vi "Initialize.vi"(7 "Serial Configuration":T1={"Baud Rate"=9600, "Flow Control"=0, "Parity"=0, "Stop Bits"=10, "Data Bits"=8} {"Stop Bits" items=["1.0"=10, "1.5"=15, "2.0"=20]; "Parity" items=["None", "Odd", "Even", "Mark", "Space"]; "Flow Control" items=["None", "XON/XOFF", "RTS/CTS"]}, 8 "error in (no error)":errorcluster, 9 "Reset (True)":bool=TRUE, 10 "ID Query (True)":bool=TRUE, 11 "VISA resource name":refnum<visa-resource-name>) -> (0 "error out":errorcluster, 3 "VISA resource name out":refnum<visa-resource-name>)   [LabVIEW 2020, in "Keithley DMM6500 DAQ6500 Series.lvlib"]
doc: "Establishes communication with the instrument and optionally performs an instrument identification query and/or an instrument reset. It also places the instrument in a default state needed for other instrument driver operations. Therefore, call this VI before calling other instrument driver VIs for this instrument. Generally, you need to call the <b>Initialize</b> VI only once at the beginning of an application."
uses:
  <instrlib>/Keithley DMM6500 DAQ6500 Series/Keithley DMM6500 DAQ6500 Series.lvlib
panel:
  # "(c) 2018-2022 National Instruments.  ALL RIGHTS RESERVED."
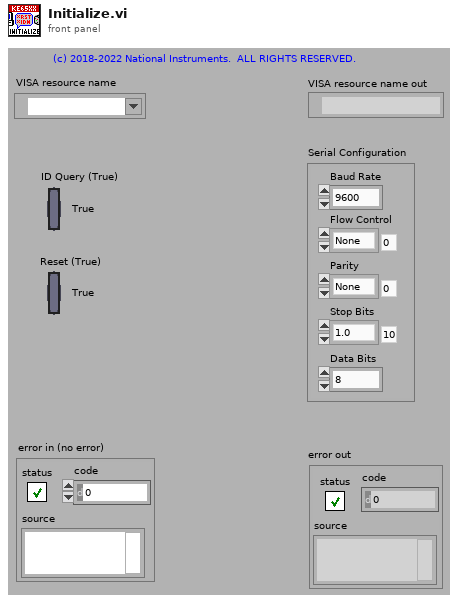
[diagram p1: front panel]
types:
  T1 = cluster{"Baud Rate":u32, "Flow Control":u16, "Parity":u16, "Stop Bits":u16, "Data Bits":u16}
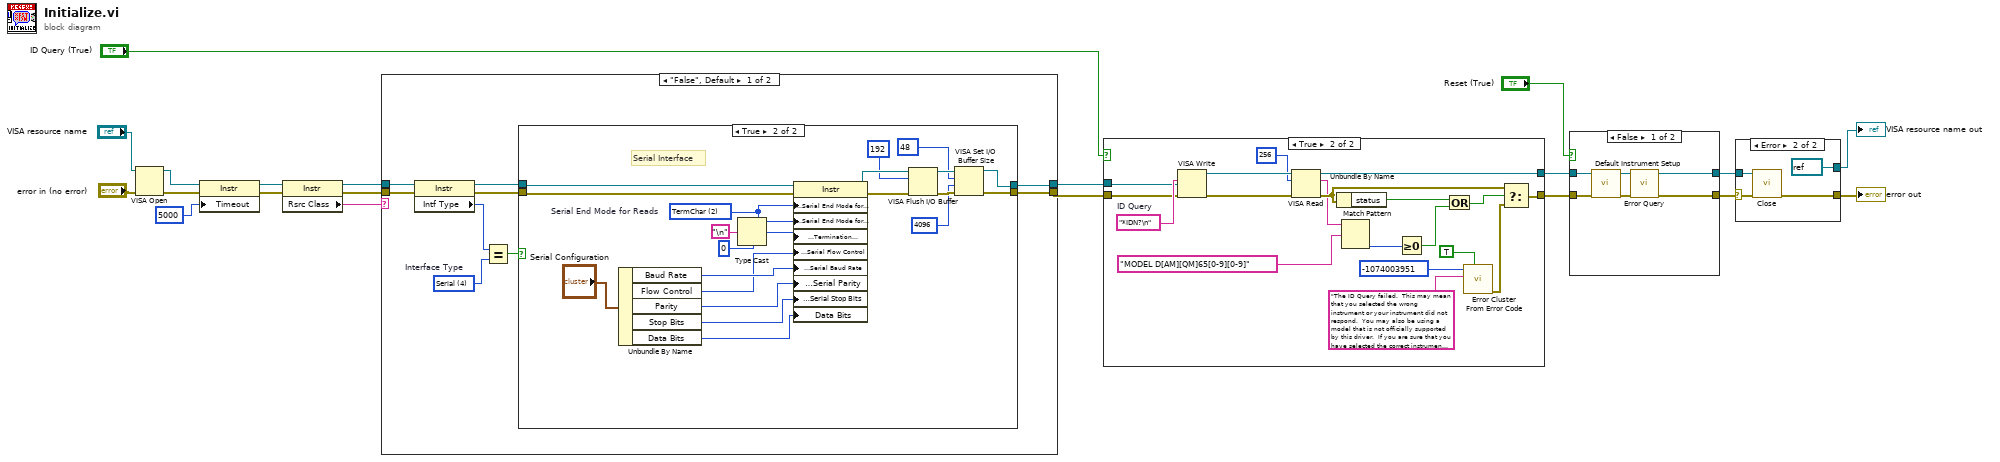
[diagram p0: block diagram]
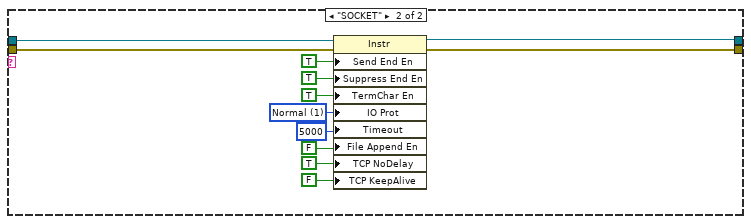
[diagram p3: hidden frame]
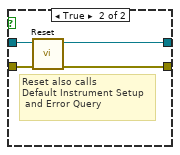
[diagram p5: hidden frame]
diagram:
  n1 = VISA Open(error in (no error)="error in (no error)", VISA resource name="VISA resource name") -> (VISA resource name=w4:refnum<visa-resource-name>, error out=w3:errorcluster)  [unwired: 3 in]
  n2 = property class="Instr"(reference=w4, error in=w3, "Timeout"=u32 5000 ("General Settings:Timeout Value")) -> (reference out=w1:refnum<visa-resource-name>, error out=w2:errorcluster)
  n3 = property class="Instr"(reference=w1, error in=w2) -> (reference out=w9:refnum<visa-resource-name>, error out=w8:errorcluster, "Rsrc Class"=w10:string)
  n4 = case shown="\"False\", Default" w10 {
    tunnel: w9 -> [w29 w61]
    tunnel: w8 -> [w28 w60]
    tunnel: [w26 w63] -> w7
    tunnel: [w25 w62] -> w6
    frame "False", Default {
      w23 = u16 4 items=["GPIB"=1, "VXI"=2, "GPIB-VXI"=3, "Serial"=4, "PXI"=5, "TCPIP"=6, "USB"=7, "FireWire"=9]  # Interface Type
      n5 = property class="Instr"(reference=w29, error in=w28) -> (reference out=w22:refnum<visa-resource-name>, error out=w27:errorcluster, "Intf Type"=w24:u16)
      n6 = Equal?(x=w24, y=w23) -> (x = y?=w21:bool)
      n7 = case shown="True" w21 {
        tunnel: w27 -> [w31 w41]
        tunnel: [w30 w40] -> w26
        tunnel: [w31 w39] -> w25
        tunnel: w22 -> [w30 w38]
        frame False {
        }
        frame True {
          w43 = u16 2 items=["None", "LastBit", "TermChar"]  # Serial End Mode for Reads
          # "Serial Interface"
          n8 = Unbundle By Name("Serial Configuration") -> ("Baud Rate"=w36:u32, "Flow Control"=w35:u16, "Parity"=w34:u16, "Stop Bits"=w33:u16, "Data Bits"=w32:u16)
          n9 = Type Cast(type=u8 0, x="\n") -> (*(type *) &x=w42:u8)
          n10 = property class="Instr"(reference=w38, error in=w41, "Serial Settings:Serial End Mode for Reads"=w43, "Serial Settings:Serial End Mode for Writes"=w43, "Message Based Settings:Termination Character"=w42, "Serial Settings:Serial Flow Control"=w35, "Serial Settings:Serial Baud Rate"=w36, "Serial Settings:Serial Parity"=w34, "Serial Settings:Serial Stop Bits"=w33, "Data Bits"=w32) -> (reference out=w49:refnum<visa-resource-name>, error out=w51:errorcluster)
          n11 = VISA Flush I/O Buffer(VISA resource name=w49, mask (16)=u16 192, error in (no error)=w51) -> (VISA resource name out=w52:refnum<visa-resource-name>, error out=w50:errorcluster)
          n12 = VISA Set I/O Buffer Size(VISA resource name=w52, mask (16)=u16 48, size (4096)=u32 4096 ("size (0)"), error in (no error)=w50) -> (VISA resource name out=w40:refnum<visa-resource-name>, error out=w39:errorcluster)
        }
      }
    }
    frame "SOCKET" {
      w56 = u16 1 items=["Normal"=1, "VXI/FDC"=2, "GPIB/HS488"=3, "Serial-TCPIP-USB/488 Strings"=4, "USBTMC/Vendor-Specific"=5] ("Message Based Settings:IO Protocol")
      n13 = property class="Instr"(reference=w61, error in=w60, "Send End En"=TRUE ("Message Based Settings:Termination Character Enable"), "Suppress End En"=TRUE ("Message Based Settings:Suppress End Enable"), "TermChar En"=TRUE ("Message Based Settings:Termination Character Enable"), "IO Prot"=w56, "Timeout"=u32 5000 ("General Settings:Timeout Value"), "File Append En"=FALSE ("Message Based Settings:File Append Enable"), "TCP NoDelay"=TRUE ("TCP/IP Settings:No Packet Delay"), "TCP KeepAlive"=FALSE ("TCP/IP Settings:Keep-Alive Packets")) -> (reference out=w63:refnum<visa-resource-name>, error out=w62:errorcluster)
    }
  }
  n14 = case shown="True" "ID Query (True)" {
    tunnel: [w65 w85] -> w19
    tunnel: [w66 w84] -> w20
    tunnel: w7 -> [w66 w68]
    tunnel: w6 -> [w65 w67]
    frame False {
    }
    frame True {
      w79 = "*IDN?\n"  # ID Query
      n15 = VISA Write(VISA resource name=w68, write buffer=w79, error in (no error)=w67) -> (VISA resource name out=w83:refnum<visa-resource-name>, error out=w82:errorcluster)  [unwired: 1 out]
      n16 = VISA Read(VISA resource name=w83, byte count=u32 256, error in (no error)=w82) -> (VISA resource name out=w84:refnum<visa-resource-name>, read buffer=w69:string, error out=w73:errorcluster)  [unwired: 1 out]
      n17 = Unbundle By Name(w73) -> ("status"=w72:bool)
      n18 = Match Pattern(string=w69, regular expression="MODEL D[AM][QM]65[0-9][0-9]") -> (offset past match=w74:i32)  [unwired: 1 in, 3 out]
      n19 = Greater Or Equal To 0?(x=w74) -> (x >= 0?=w71:bool)
      n20 = Or(x=w72, y=w71) -> (x .or. y?=w70:bool)
      n21 = call <vilib>:"Error Cluster From Error Code.vi"("show call chain? (False)"=TRUE, "error message (\"\")"="The ID Query failed.  This may mean that you selected the wrong instrument or your instrument did not respond.  You may also be using a model that is not officially supported by this driver.  If you are sure that you have selected the correct instrument and it is responding, try disabling the ID Query." ("Source (VI Name)"), "error code (0)"=-1074003951 ("Code")) -> ("error out"=w78:errorcluster)  [unwired: 6 in]
      n22 = Select(t=w73, s=w70, f=w78) -> (s? t:f=w85:errorcluster)
    }
  }
  n23 = case shown="False" "Reset (True)" {
    tunnel: w19 -> [w90 w92]
    tunnel: [w87 w95] -> w11
    tunnel: w20 -> [w91 w93]
    tunnel: [w88 w94] -> w12
    frame False {
      n24 = call <instrlib>:"Default Instrument Setup.vi"("error in (no error)"=w90, "VISA resource name"=w91) -> ("error out"=w86:errorcluster, "VISA resource name out"=w89:refnum<visa-resource-name>)  [unwired: 8 in]
      n25 = call <instrlib>:"Error Query.vi"("error in (no error)"=w86, "VISA resource name"=w89) -> ("error out"=w87:errorcluster, "VISA resource name out"=w88:refnum<visa-resource-name>)  [unwired: 6 in, 2 out]
    }
    frame True {
      # "Reset also calls \nDefault Instrument Setup\n and Error Query"
      n26 = call <instrlib>:"Reset.vi"("error in (no error)"=w92, "VISA resource name"=w93) -> ("error out"=w95:errorcluster, "VISA resource name out"=w94:refnum<visa-resource-name>)  [unwired: 8 in]
    }
  }
  n27 = case shown="Error" w11 {
    selector: w11 -> [w96 w99]
    tunnel: w12 -> [w97 w100]
    tunnel: [w97 refnum<visa-resource-name> refnum ("VISA resource name out")] -> w14
    tunnel: [w96 w101] -> w13
    frame No Error {
    }
    frame Error {
      n28 = call <instrlib>:"Close.vi"("error in (no error)"=w99, "VISA resource name"=w100) -> ("error out"=w101:errorcluster)  [unwired: 9 in]
    }
  }
  "VISA resource name out" <- w14
  "error out" <- w13
